vi "Timed_DeBounce.vi"(1 "Input":bool, 2 "Reset":bool, 3 "Hold Time(ms)":u32) -> (0 "Output":bool)   [LabVIEW 2017, in "ArgosLib.lvlib"]
uses:
  TypeDefs/EdgeDetector_Type.ctl
  ArgosLib.lvlib
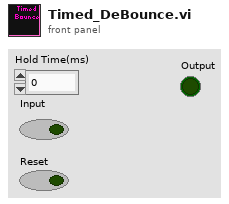
[diagram p1: front panel]
types:
  T1 = typedef "ArgosLib.lvlib/EdgeDetector_Type.ctl" = enum16{"RisingEdge", "FallingEdge", "Both"}
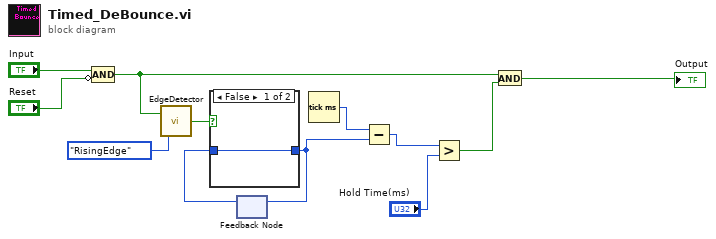
[diagram p0: block diagram]
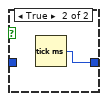
[diagram p2: hidden frame]
diagram:
  n1 = Compound Arithmetic op=AND("Input", invert "Reset") -> (w2:bool)
  n2 = call "EdgeDetector.vi"("DetectorType"=EdgeDetector_Type."RisingEdge", "Input"=w2) -> ("Edge"=w9:bool)
  n3 = feedback #1() -> (w6:u32)  [unwired: 1 in]
  n4 = case shown="False" w9 {
    tunnel: [w13 w14] -> w5
    tunnel: w6 -> [w13 _]
    frame False {
    }
    frame True {
      n5 = Tick Count (ms)() -> (millisecond timer value=w14:u32)
    }
  }
  n6 = feedback-in #1(w5) -> ()
  n7 = Tick Count (ms)() -> (millisecond timer value=w10:u32)
  n8 = Subtract(x=w10, y=w5) -> (x-y=w11:u32)
  n9 = Greater?(x=w11, y="Hold Time(ms)") -> (0:w12:bool)
  n10 = And(x=w2, y=w12) -> (x .and. y?=→"Output":bool)
